vi "Return Home.vi"(6 "chip select  (1st chip)":enum16{"1st chip", "2nd chip"}(ring), 8 "error in (no error)":errorcluster, 11 "HD44780 in":refnum<class "HD44780.lvclass">) -> (0 "error out":errorcluster, 3 "HD44780 out":refnum<class "HD44780.lvclass">)   [LabVIEW 2017, in "HD44780.lvclass"]
uses:
  HD44780.lvclass
  HD44780.lvclass/HD44780.ctl
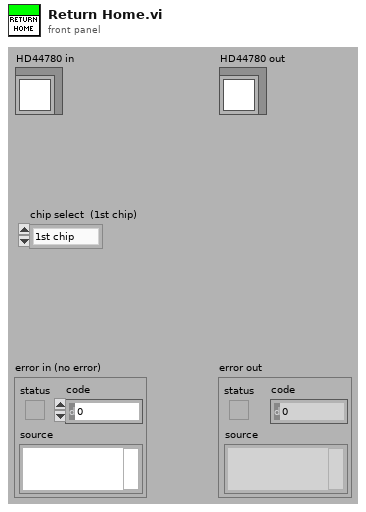
[diagram p1: front panel]
types:
  T1 = typedef "HD44780 Common.lvlib/cluster of class private data.ctl" = cluster{"FPGA VI Reference":refnum<k20>, "device index":i8, "screen size":T2, "font size":T3, "auto wrap":bool, "alignment":T4, "number of line":T5, "shift 0":i8, "entry mode 0":T6, "shift 1":i8, "entry mode 1":T6}
  T2 = typedef "HD44780 Common.lvlib/screen size.ctl" = enum8{"8x1", "8x2", "12x4", "16x1", "16x2", "16x4", "20x1", "20x2", "20x4", "24x1", "24x2", "40x2", "40x4"}
  T3 = typedef "HD44780 Common.lvlib/font size.ctl" = enum8{"5x8", "5x10"}
  T4 = typedef "HD44780 Common.lvlib/alignment.ctl" = enum16{"None", "Left", "Center", "Right"}
  T5 = typedef "HD44780 Common.lvlib/line number.ctl" = enum8{"1 line", "2 lines"}
  T6 = typedef "HD44780 Common.lvlib/entry mode.ctl" = enum8{"increment & no shift", "increment & shift", "decrement & no shift", "decrement & shift"}
  T7 = cluster{"FPGA VI Reference":refnum<k20>, "device index":i8, "screen size":enum8{"8x1", "8x2", "12x4", "16x1", "16x2", "16x4", "20x1", "20x2", "20x4", "24x1", "24x2", "40x2", "40x4"}, "font size":enum8{"5x8", "5x10"}, "auto wrap":bool, "alignment":enum16{"None", "Left", "Center", "Right"}, "number of line":enum8{"1 line", "2 lines"}, "shift 0":i8, "entry mode 0":enum8{"increment & no shift", "increment & shift", "decrement & no shift", "decrement & shift"}, "shift 1":i8, "entry mode 1":enum8{"increment & no shift", "increment & shift", "decrement & no shift", "decrement & shift"}}
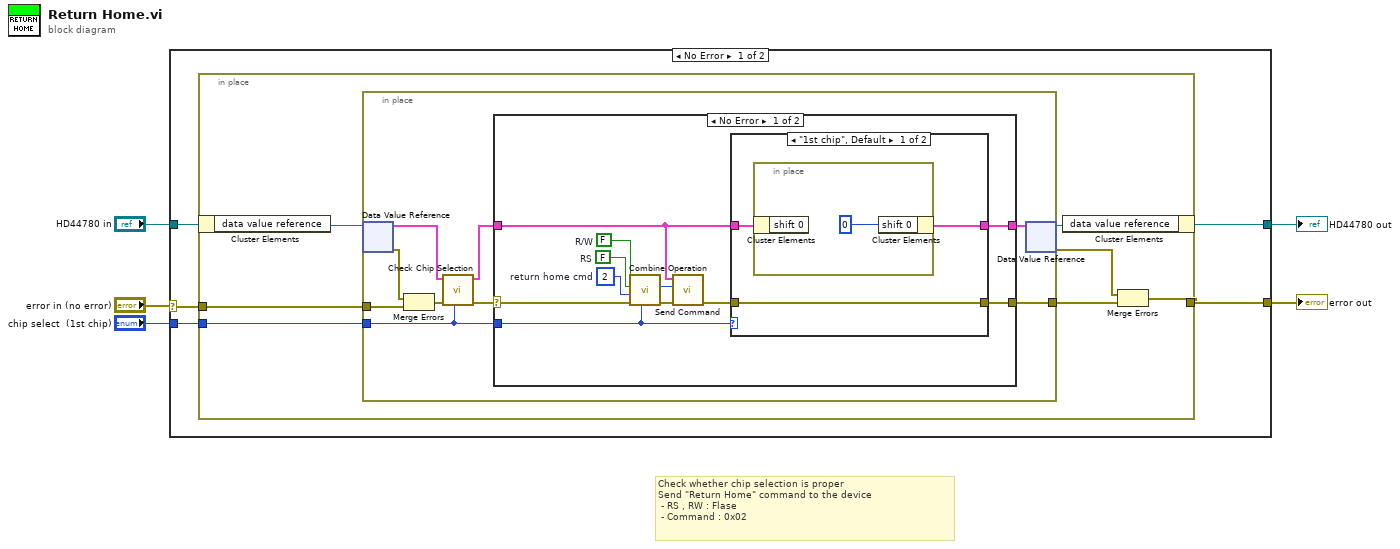
[diagram p0: block diagram]
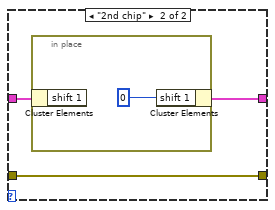
[diagram p2: hidden frame]
diagram:
  # "Check whether chip selection is proper\nSend \"Return Home\" command to the device\n - RS , RW : Flase\n - Command : 0x02"
  n1 = case shown="No Error" "error in (no error)" {
    selector: "error in (no error)" -> [w6 w48]
    tunnel: [w10 w48] -> w5
    tunnel: "chip select  (1st chip)" -> [w9 _]
    tunnel: "HD44780 in" -> [w8 w49]
    tunnel: [w7 w49] -> w1
    frame No Error {
      n2 = in-place {
        in-place-border: [w11] -> w10
        in-place-border: w9 -> [w17]
        in-place-border: w6 -> [w14]
        n3 = in-place-cluster #1(w8) -> ("data value reference"=w16:refnum<data-value>)
        n4 = in-place {
          in-place-border: [w26] -> w12
          in-place-border: w17 -> [w18]
          in-place-border: w14 -> [w23]
          n5 = in-place-dvr #2(w16) -> (w20:T1, w24:errorcluster)
          n6 = Merge Errors(w24, w23) -> (w22:errorcluster)
          n7 = call "Check Chip Selection.vi"("chip select"=w18, "error in (no error)"=w22, "cluster of private data in"=w20) -> ("error out"=w21:errorcluster, "cluster of private data out"=w19:T7)  [unwired: 7 in]
          n8 = case shown="No Error" w21 {
            selector: w21 -> [w29 w47]
            tunnel: [w32 w47] -> w26
            tunnel: w19 -> [w28 w46]
            tunnel: [w33 w46] -> w25
            tunnel: w18 -> [w27 _]
            frame No Error {
              w30 = FALSE  # RS
              w37 = u8 2  # return home cmd
              w31 = FALSE  # R/W
              n9 = call "Combine Operation.vi"("chip select  (1st chip)"=w27, "error in (no error)"=w29, "cmd/data"=w37, "RS"=w30, "R/W"=w31) -> ("error out"=w36:errorcluster, "output"=w34:u32)  [unwired: 5 in]
              n10 = call "Send Command.vi"("error in (no error)"=w36, "operation"=w34, "cluster of private data in"=w28) -> ("error out"=w35:errorcluster)  [unwired: 6 in, 2 out]
              n11 = case shown="\"1st chip\", Default" w27 {
                tunnel: w35 -> [w38 w42]
                tunnel: w28 -> [w40 w44]
                tunnel: [w39 w43] -> w33
                tunnel: [w38 w42] -> w32
                frame "1st chip", Default {
                  n12 = in-place {
                    n13 = in-place-cluster #3(w40) -> ()  [unwired: 1 out]
                    n14 = in-place-cluster #3("shift 0"=i8 0 ("shift 1")) -> (w39:T7)
                  }
                }
                frame "2nd chip" {
                  n15 = in-place {
                    n16 = in-place-cluster #4(w44) -> ()  [unwired: 1 out]
                    n17 = in-place-cluster #4("shift 1"=i8 0) -> (w43:T7)
                  }
                }
              }
            }
            frame Error {
            }
          }
          n18 = in-place-dvr #2(w25) -> (w15:refnum<data-value>, w13:errorcluster)
        }
        n19 = in-place-cluster #1("data value reference"=w15) -> (w7:refnum<class "HD44780.lvclass">)
        n20 = Merge Errors(w13, w12) -> (w11:errorcluster)
      }
    }
    frame Error {
    }
  }
  "error out" <- w5
  "HD44780 out" <- w1
